vi "filter tags by readers.vi"(9 "include? (default: exclude)":bool, 10 "reader modules":string[](array[string]), 11 "engine configuration in":refnum<class "engine configuration.lvclass">) -> (2 "tag list":refnum<class "tag descriptor.lvclass">[](array[class]), 3 "engine configuration out":refnum<class "engine configuration.lvclass">)   [LabVIEW 2013, in "engine configuration.lvclass"]
doc: "This function returns a list of tags that either have one of the 'reader modules' listed as a reader (include) or that don't have one of the 'reader modules' listed as a reader (exclude)."
uses:
  engine configuration.lvclass
  <vilib>/NI/Tag Bus/tag/tag descriptor.lvclass
  engine configuration.lvclass/engine configuration.ctl
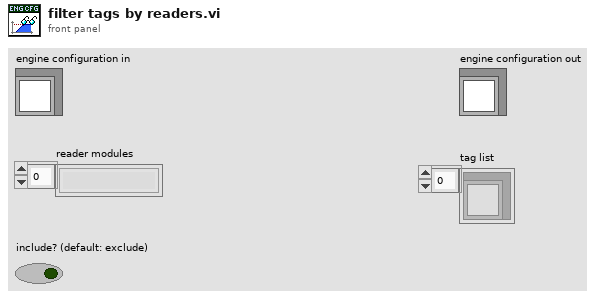
[diagram p1: front panel]
types:
  T1 = typedef "engine configuration.lvclass/module channel pairings.ctl" = cluster{"modules":string[], "channels":string[]}
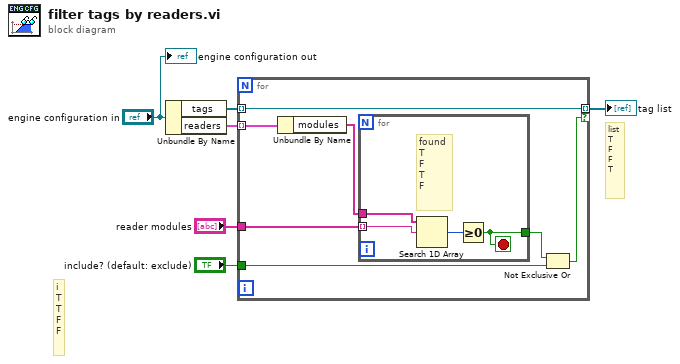
[diagram p0: block diagram]
diagram:
  # "list\nT\nF\nF\nT"
  # "i\nT\nT\nF\nF"
  n1 = Unbundle By Name("engine configuration in") -> ("tags"=w2:refnum<class "tag descriptor.lvclass">[], "readers"=w1:T1[])
  n2 = for {
    tunnel: [w9] -> w5 mode=indexing if=w10
    tunnel: "reader modules" -> [w13]
    tunnel: "include? (default: exclude)" -> [w11]
    tunnel: w2 -> [w9] mode=indexing
    tunnel: w1 -> [w8] mode=indexing
    n3 = Unbundle By Name(w8) -> ("modules"=w7:string[])
    n4 = for {
      tunnel: w13 -> [w16] mode=indexing
      tunnel: w7 -> [w15]
      tunnel: [w14] -> w12
      stop <- w14 stop-if-true
      # "found\nT\nF\nT\nF"
      n5 = Search 1D Array(1D array=w15, element=w16) -> (index of element=w17:i32)  [unwired: 1 in]
      n6 = Greater Or Equal To 0?(x=w17) -> (x >= 0?=w14:bool)
    }
    n7 = Not Exclusive Or(1:w11, 2:w12) -> (0:w10:bool)
  }
  "tag list" <- w5
  "engine configuration out" <- "engine configuration in"
